vi "test_tilt_stage_positions.vi"() -> ()   [LabVIEW 2016]
uses:
  <vilib>/measure/madcrms.llb/Averaged DC-RMS for 1 Chan.vi
  <instrlib>/Agilent 2000 3000 X-Series/Agilent 2000 3000 X-Series.lvlib
  <vilib>/measure/NI_MAPro.lvlib
panel:
  in  "Steps":i32=200
  in  "file path (use dialog)":path=path "C:/Users/UsphereLab/Documents/LabVIEW Data/axis_motor_and_voltage.txt"
  out "error out 2":errorcluster
  out "Waveform Data 2":waveform(dbl)[](graph)
  out "Waveform Data":dbl[](graph)
  out "End Waveform":i32(graph)
  in  "#repeats":i32=10
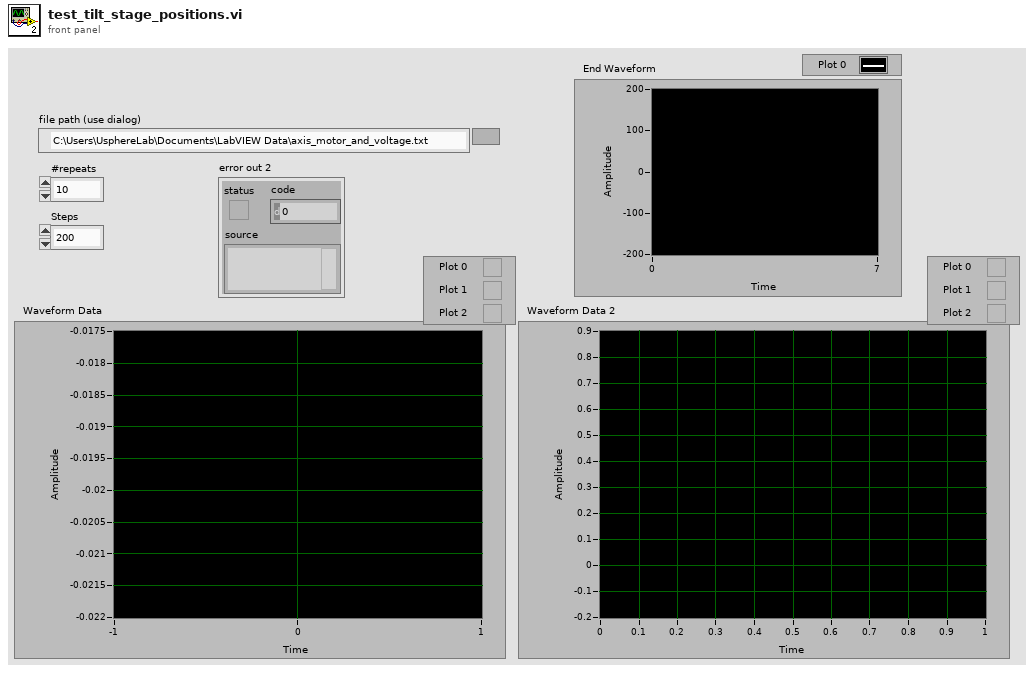
[diagram p1: front panel]
types:
  T1 = enum16{"open", "replace", "create", "open or create", "replace or create", "replace or create with confirmation"}
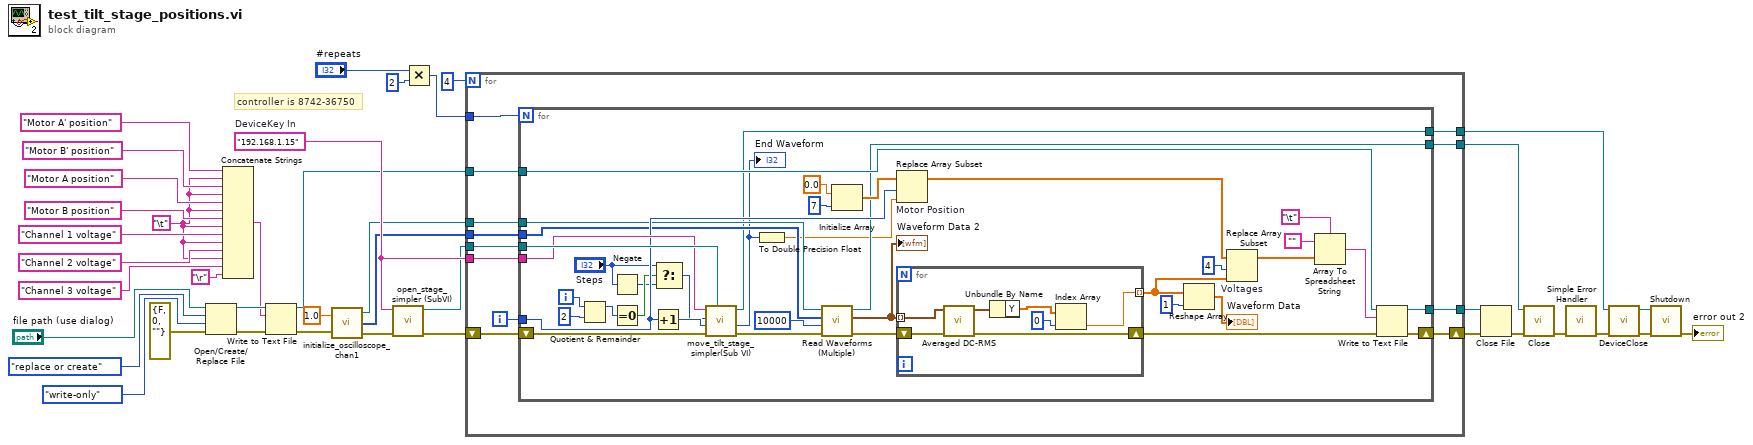
[diagram p0: block diagram]
diagram:
  w33 = "192.168.1.15"  # DeviceKey In
  w17 = "\t"
  # "controller is 8742-36750"
  n1 = Open/Create/Replace File(file path (use dialog)="file path (use dialog)", error in=errorcluster {"status"=FALSE, "code"=0, "source"=""} ("error in (no error)"), operation (0:open)=T1."replace or create", access (0:read/write)=enum16{"read/write", "read-only", "write-only"}."write-only") -> (refnum out=w24:refnum<file>, error out=w25:errorcluster)  [unwired: 2 in, 1 out]
  n2 = Concatenate Strings("Motor A' position" ("string"), w17, "Motor B' position" ("string"), w17, "Motor A position" ("string"), w17, "Motor B position" ("string"), w17, "Channel 1 voltage" ("string"), w17, "Channel 2 voltage" ("string"), w17, "Channel 3 voltage" ("string"), "\r") -> (w23:string)
  n3 = Write to Text File(file (use dialog)=w24, text=w23, error in=w25) -> (refnum out=w26:refnum<file>, error out=w3:errorcluster)  [unwired: 1 in, 1 out]
  n4 = call "initialize_oscilloscope_chan1.vi"("Range (0.001 S)"=1.0, "error in (no error)"=w3) -> ("VISA resource name out"=w13:refnum<visa-resource-name>, "channels"=w14:i32[], "error out"=w2:errorcluster)
  n5 = call "open_stage_simpler (SubVI).vi"("error in (no error)"=w2, "IP address"=w33) -> ("error out"=w1:errorcluster, "reference"=w22:refnum<k24>)  [unwired: 7 in, 1 out]
  n6 = Multiply(x="#repeats", y=2) -> (x*y=w20:i32)
  n7 = for {
    N: 4 -> [_]
    shift-right: [w49] -> w39
    shift-left: w1 -> [w50]
    tunnel: w26 -> [w51]
    tunnel: [w48] -> w38
    tunnel: w33 -> [w47]
    tunnel: w20 -> [w46]
    tunnel: w22 -> [w45]
    tunnel: w14 -> [w43]
    tunnel: w13 -> [w42]
    tunnel: [w41] -> w11
    tunnel: [w40] -> w8
    i -> [w44]
    n8 = for {
      N: w46 -> [_]
      tunnel: w44 -> [w78]
      tunnel: w47 -> [w83]
      shift-right: [w87] -> w49
      shift-left: w50 -> [w54]
      tunnel: w51 -> [w89]
      tunnel: [w86] -> w48
      tunnel: w45 -> [w84]
      tunnel: w43 -> [w62]
      tunnel: w42 -> [w61]
      tunnel: [w60] -> w41
      tunnel: [w58] -> w40
      i -> [w74]
      n9 = Quotient & Remainder(x=w74, y=2) -> (x-y*floor(x/y)=w72:i32)  [unwired: 1 out]
      n10 = Negate(x="Steps") -> (-x=w69:i32)
      n11 = Equal To 0?(x=w72) -> (x = 0?=w71:bool)
      n12 = Increment(x=w78) -> (x+1=w79:i32)
      n13 = Select(t="Steps", s=w71, f=w69) -> (s? t:f=w68:i32)
      n14 = call "move_tilt_stage_simpler(Sub VI).vi"(".NET Refnum in"=w84, "error in (no error)"=w54, "motor"=w79, "relativeSteps"=w68, "deviceKey"=w83) -> ("error out"=w63:errorcluster, "End position"=w52:i32, ".NET Refnum out"=w58:refnum<k24>)  [unwired: 1 out]
      "End Waveform" <- w52
      n15 = To Double Precision Float(number=w52) -> (double precision float=w53:dbl)
      n16 = call <instrlib>:"Read Waveforms (Multiple).vi"("error in (no error)"=w63, "Timeout (10000 ms)"=u32 10000 ("Maximum Time (10000 ms)"), "Channels"=w62, "VISA resource name"=w61) -> ("error out"=w56:errorcluster, "Waveform Data"=w64:waveform(dbl)[], "VISA resource name out"=w60:refnum<visa-resource-name>)  [unwired: 5 out]
      "Waveform Data 2" <- w64
      n17 = Initialize Array(0.0 ("element"), 7 ("dimension size")) -> (w80:dbl[])
      n18 = Replace Array Subset "Motor Position"(array=w80, new element=w53, index=w78) -> (w76:dbl[])
      n19 = for {
        tunnel: w64 -> [w94] mode=indexing
        tunnel: [w92] -> w59 mode=indexing
        shift-right: [w90] -> w55
        shift-left: w56 -> [w91]
        n20 = call-poly <vilib>:"Averaged DC-RMS.vi"("error in (no error)"=w91, "signal in"=w94) -> ("error out"=w90:errorcluster, "DC value waveform"=w93:waveform(dbl))  [unwired: 5 in, 3 out]
        n21 = Unbundle By Name(w93) -> ("Y"=w96:dbl[])
        n22 = Index Array "Index Array"(array=w96, index=0) -> (element=w92:dbl)
      }
      n23 = Reshape Array(w59, 1 ("dimension size")) -> (→"Waveform Data":dbl[])
      n24 = Replace Array Subset "Voltages"(array=w76, new element=w59, index=4) -> (w67:dbl[])
      n25 = Array To Spreadsheet String(delimiter (Tab)="\t", array=w67, 3:"") -> (spreadsheet string=w88:string)
      n26 = Write to Text File(file (use dialog)=w89, text=w88, error in=w55) -> (refnum out=w86:refnum<file>, error out=w87:errorcluster)  [unwired: 1 in, 1 out]
    }
  }
  n27 = Close File(refnum=w38, error in=w39) -> (error out=w5:errorcluster)  [unwired: 1 out]
  n28 = call <instrlib>:"Close.vi"("error in (no error)"=w5, "VISA resource name"=w11) -> ("error out"=w12:errorcluster)  [unwired: 9 out]
  n29 = call <vilib>:"Simple Error Handler.vi"("error in (no error)"=w12) -> ("error out"=w7:errorcluster)  [unwired: 1 in, 7 out]
  n30 = call "DeviceClose.vi"("error in (no error)"=w7, "CmdLib In"=w8) -> ("error out"=w9:errorcluster, "CmdLib Out"=w10:refnum<k24>)  [unwired: 3 in, 1 out]
  n31 = call "Shutdown.vi"("error in (no error)"=w9, "CmdLib In"=w10) -> ("error out"=→"error out 2":errorcluster)  [unwired: 4 in, 1 out]
